vi "Write Tree.vi"(8 "error in (no error)":errorcluster, 10 "Tree":T1(array[cluster]), 11 "Fast Tree in":refnum<class "Fast Tree.lvclass">) -> (0 "error out":errorcluster, 3 "Fast Tree out":refnum<class "Fast Tree.lvclass">)   [LabVIEW 2019, in "Fast Tree.lvclass"]
uses:
  Fast Tree.lvclass
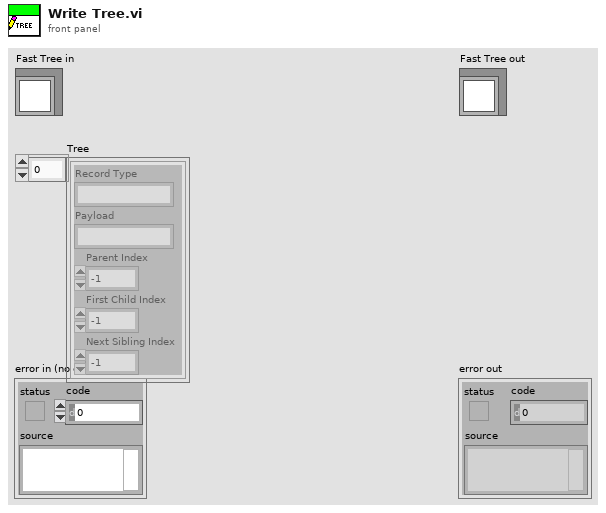
[diagram p1: front panel]
types:
  T1 = cluster{"Record Type":string, "Payload":string, "Parent Index":i32, "First Child Index":i32, "Next Sibling Index":i32}[]
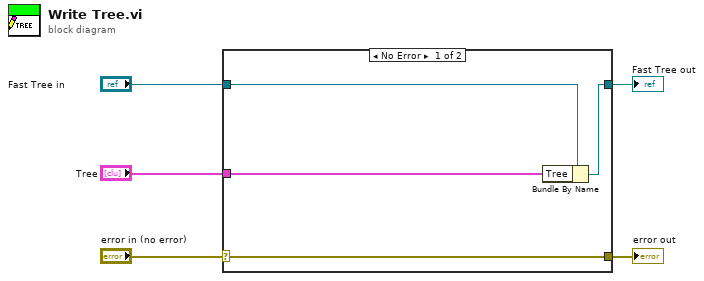
[diagram p0: block diagram]
diagram:
  n1 = case shown="No Error" "error in (no error)" {
    selector: "error in (no error)" -> [w9 w10]
    tunnel: [w9 w10] -> w4
    tunnel: [w7 w11] -> w2
    tunnel: "Fast Tree in" -> [w8 w11]
    tunnel: "Tree" -> [w6 _]
    frame No Error {
      n2 = Bundle By Name(cluster=w8, "Tree"=w6) -> (w7:refnum<class "Fast Tree.lvclass">)
    }
    frame Error {
    }
  }
  "error out" <- w4
  "Fast Tree out" <- w2
